vi "REQ Get Username.vi"(6 "wait for reply (T)":bool=TRUE, 8 "error in":errorcluster, 10 "User Level":enum16{"Administrator", "Engineer", "Operator"}(ring)) -> (0 "error out":errorcluster, 1 "timed out?":bool, 3 "Username":string[](array[string]))   [LabVIEW 2016, in "Database.lvlib"]
doc: "_____\nCreated using DQMH Event Scripter 7.0.0.1280."
uses:
  Database.lvlib
  REQ Get Username Argument--cluster.ctl
  REQ Get Username (Reply Payload)--cluster.ctl
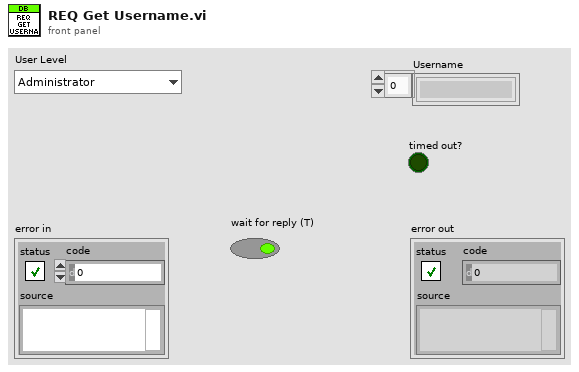
[diagram p1: front panel]
types:
  T1 = typedef "Database.lvlib/REQ Get Username Argument--cluster.ctl" = cluster{"User Level":enum16{"Administrator", "Engineer", "Operator"}, "Wait Notifier":refnum<notifier>, "wait for reply":bool}
  T2 = typedef "Database.lvlib/Request Events--cluster.ctl" = cluster{"Stop Module":refnum<user-event>, "Show Panel":refnum<user-event>, "Hide Panel":refnum<user-event>, "Get Module Execution Status":refnum<user-event>, "Show Diagram":refnum<user-event>, "REQ Add User":refnum<user-event>, "REQ Check Credential":refnum<user-event>, "REQ Delete User":refnum<user-event>, "REQ Update User Details":refnum<user-event>, "REQ List Table":refnum<user-event>, "REQ Delete Table Data":refnum<user-event>, "REQ Save DB Record Data":refnum<user-event>, "REQ Save Test Data":refnum<user-event>, "REQ Load Test Data":refnum<user-event>, "REQ Get Username":refnum<user-event>, "REQ Close DB Ref":refnum<user-event>, "REQ Retry DB":refnum<user-event>, "REQ DB Setup":refnum<user-event>, "REQ Write Test Info":refnum<user-event>, "REQ Fetch Coulmn Name":refnum<user-event>}
  T3 = typedef "Database.lvlib/REQ Get Username (Reply Payload)--cluster.ctl" = cluster{"Username":string[], "error":errorcluster}
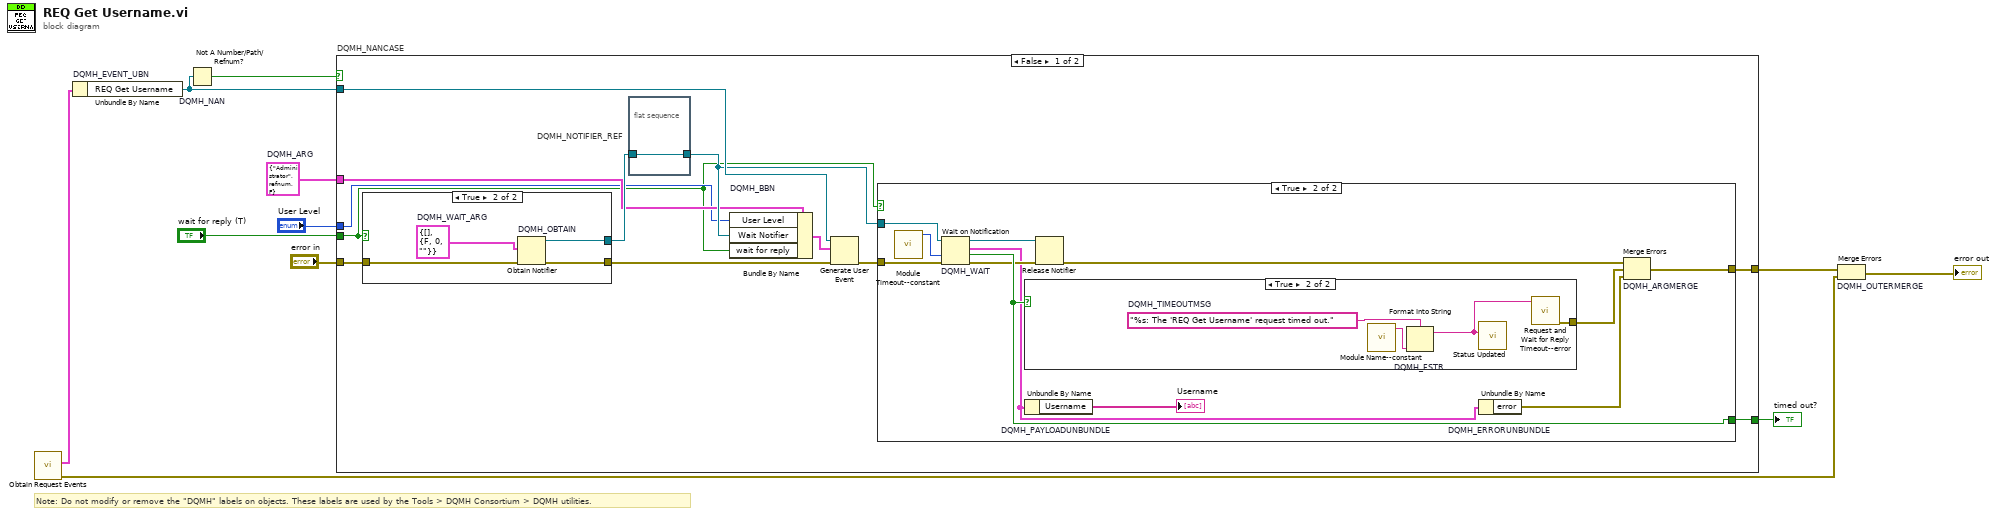
[diagram p0: block diagram]
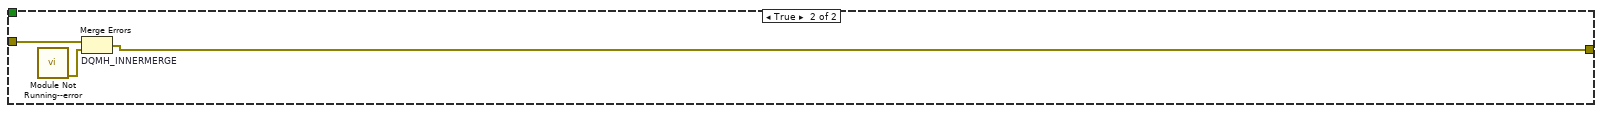
[diagram p5: hidden frame]
diagram:
  w5 = T1 {"User Level"=enum."Administrator", "Wait Notifier"=refnum, "wait for reply"=FALSE}  # DQMH_ARG
  # "Note: Do not modify or remove the \"DQMH\" labels on objects. These labels are used by the Tools > DQMH Consortium > DQMH utilities."
  n1 = call "Obtain Request Events.vi"() -> ("error out"=w2:errorcluster, "Database Request Events"=w1:T2)  [unwired: 10 in]
  n2 = Unbundle By Name "DQMH_EVENT_UBN"(w1) -> ("REQ Get Username"=w9:refnum<user-event>)
  n3 = Not A Number/Path/Refnum? "DQMH_NAN"(number/path/refnum=w9) -> (NaN/Path/Refnum?=w8:bool)
  n4 = case "DQMH_NANCASE" shown="False" w8 {
    tunnel: "error in" -> [w23 w49]
    tunnel: w9 -> [w21 _]
    tunnel: [w18 w48] -> w6
    tunnel: [w19 _] -> w7
    tunnel: w5 -> [w14 _]
    tunnel: "User Level" -> [w13 _]
    tunnel: "wait for reply (T)" -> [w12 _]
    frame False {
      n5 = case shown="True" w12 {
        tunnel: w23 -> [w42 w46]
        tunnel: [w42 w45] -> w20
        tunnel: [_ w43] -> w16
        frame False {
        }
        frame True {
          w44 = T3 {"Username"=[], "error"={"status"=FALSE, "code"=0, "source"=""}}  # DQMH_WAIT_ARG
          n6 = Obtain Notifier "DQMH_OBTAIN"(notification data type=w44, error in (no error)=w46) -> (notifier out=w43:refnum<notifier>, error out=w45:errorcluster)  [unwired: 2 in, 1 out]
        }
      }
      n7 = flat-sequence "DQMH_NOTIFIER_REF" {
        tunnel: w16 -> [w24]
        tunnel: [w24] -> w15
        frame #0 {
        }
      }
      n8 = Bundle By Name "DQMH_BBN"(cluster=w14, "User Level"=w13, "Wait Notifier"=w15, "wait for reply"=w12) -> (w17:T1)
      n9 = Generate User Event(user event=w21, event data cluster=w17, error in=w20) -> (error out=w22:errorcluster)  [unwired: 1 in, 1 out]
      n10 = case shown="True" w12 {
        tunnel: w22 -> [w25 w37]
        tunnel: w15 -> [_ w36]
        tunnel: [_ w34] -> w19
        tunnel: [w25 w33] -> w18
        frame False {
        }
        frame True {
          n11 = call "Module Timeout--constant.vi"() -> ("Module Timeout"=w27:i32)  [unwired: 11 in]
          n12 = Wait on Notification "DQMH_WAIT"(notifier=w36, timeout in ms (-1)=w27, error in (no error)=w37) -> (notifier out=w35:refnum<notifier>, notification=w28:T3, timed out?=w34:bool, error out=w32:errorcluster)  [unwired: 1 in]
          n13 = case shown="True" w34 {
            tunnel: [_ w39] -> w29
            frame False {
            }
            frame True {
              w41 = "%s: The 'REQ Get Username' request timed out."  # DQMH_TIMEOUTMSG
              n14 = call "Module Name--constant.vi"() -> ("Module Name"=w38:string)  [unwired: 11 in]
              n15 = Format Into String "DQMH_FSTR"(format string=w41, w38) -> (resulting string=w40:string)  [unwired: 2 in, 1 out]
              n16 = call "Status Updated.vi"("Status"=w40) -> ()  [unwired: 10 in, 1 out]
              n17 = call "Request and Wait for Reply Timeout--error.vi"("Error Message"=w40) -> ("error out"=w39:errorcluster)  [unwired: 10 in]
            }
          }
          n18 = Unbundle By Name "DQMH_PAYLOADUNBUNDLE"(w28) -> ("Username"=→"Username":string[])
          n19 = Release Notifier(notifier=w35, error in (no error)=w32) -> (error out=w31:errorcluster)  [unwired: 1 in, 2 out]
          n20 = Unbundle By Name "DQMH_ERRORUNBUNDLE"(w28) -> ("error"=w30:errorcluster)
          n21 = Merge Errors "DQMH_ARGMERGE"(w31, w29, w30) -> (w33:errorcluster)
        }
      }
    }
    frame True {
      n22 = call "Module Not Running--error.vi"() -> ("error out"=w47:errorcluster)  [unwired: 11 in]
      n23 = Merge Errors "DQMH_INNERMERGE"(w49, w47) -> (w48:errorcluster)
    }
  }
  "timed out?" <- w7
  n24 = Merge Errors "DQMH_OUTERMERGE"(w6, w2) -> (→"error out":errorcluster)
